vi "Flush Queue to File.vi"(8 "error in (no error)":errorcluster, 11 "Event Reporter Module in":refnum<class "Event Reporter Module.lvclass">) -> (0 "error out":errorcluster, 3 "Event Reporter Module out":refnum<class "Event Reporter Module.lvclass">)   [LabVIEW 2020, in "Volatus.lvlib" / "Event Reporter Module.lvclass"]
uses:
  Event Reporter Module.lvclass
  Event Reporter Module.lvclass/Event Reporter Module.ctl
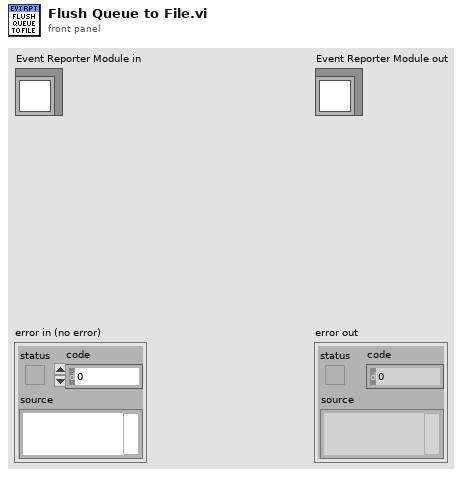
[diagram p1: front panel]
types:
  T1 = typedef "Volatus.lvlib/Event.ctl" = cluster{"Time Stamp":timestamp, "Event Level":T2, "Context":string, "Message":string, "Error":errorcluster}
  T2 = typedef "Volatus.lvlib/Event Level.ctl" = enum16{"Debug", "Info", "Warning", "Error"}
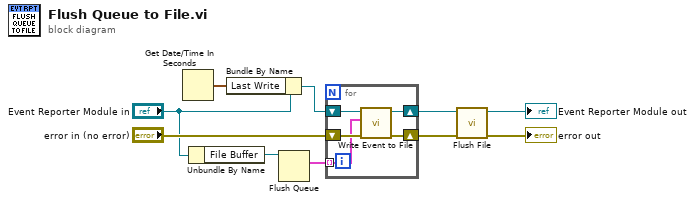
[diagram p0: block diagram]
diagram:
  n1 = Get Date/Time In Seconds() -> (seconds since 1Jan1904=w4:timestamp)
  n2 = Unbundle By Name("Event Reporter Module in") -> ("File Buffer"=w9:refnum<queue>)
  n3 = Bundle By Name(cluster="Event Reporter Module in", "Last Write"=w4) -> (w5:refnum<class "Event Reporter Module.lvclass">)
  n4 = Flush Queue(queue=w9) -> (remaining elements=w7:T1[])  [unwired: 1 in, 2 out]
  n5 = for {
    shift-right: [w12] -> w2
    shift-left: w5 -> [w15]
    shift-right: [w11] -> w6
    shift-left: "error in (no error)" -> [w14]
    tunnel: w7 -> [w13] mode=indexing
    n6 = call "Write Event to File.vi"("error in (no error)"=w14, "Event"=w13, "Event Reporter Module in"=w15) -> ("error out"=w11:errorcluster, "Event Reporter Module out"=w12:refnum<class "Event Reporter Module.lvclass">)  [unwired: 7 in]
  }
  n7 = call "Flush File.vi"("error in (no error)"=w6, "Event Reporter Module in"=w2) -> ("error out"=→"error out":errorcluster, "Event Reporter Module out"=→"Event Reporter Module out":refnum<class "Event Reporter Module.lvclass">)  [unwired: 8 in]
